vi "Delete row.vi"(10 "tetris block":u8[][](array[numeric])) -> (0 "Rows Deleted":u16, 2 "new tetris block":u8[][](array[numeric]))   [LabVIEW 2018]
panel:
  out "error out":errorcluster
  in  "error in (no error)":errorcluster
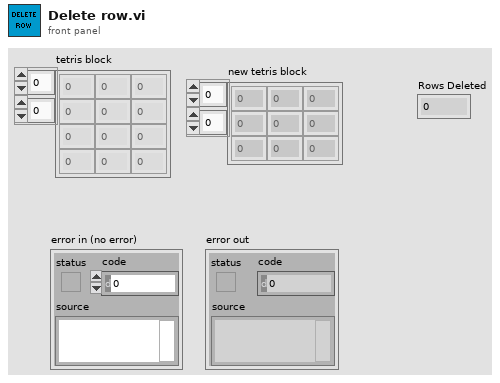
[diagram p1: front panel]
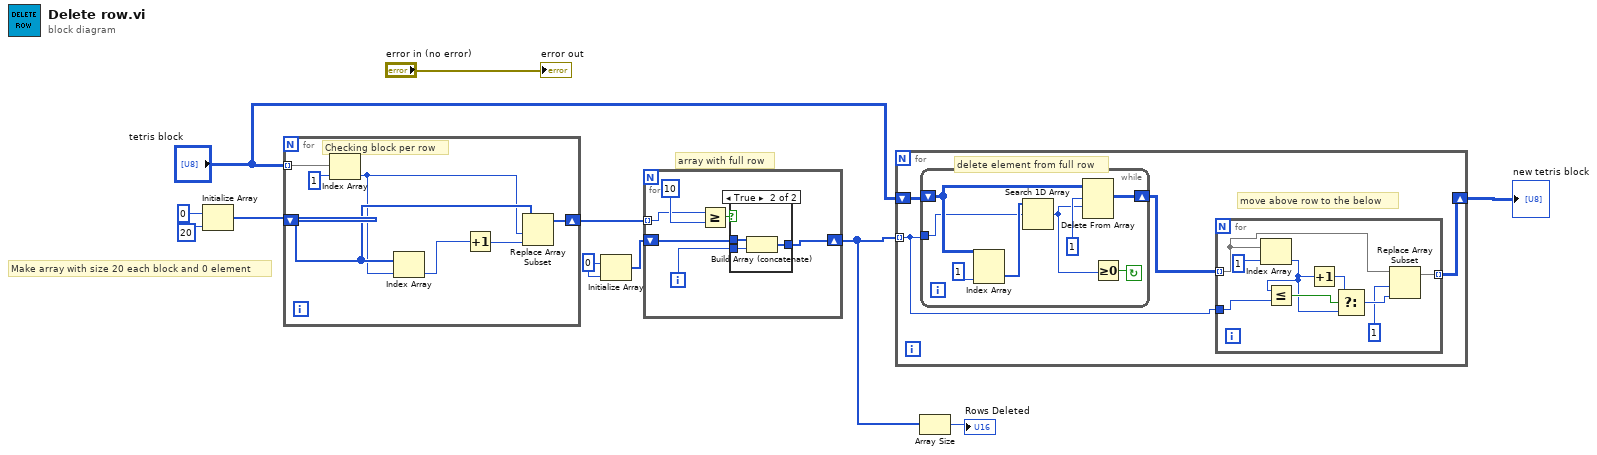
[diagram p0: block diagram]
diagram:
  w5 = 0
  # "array with full row"
  # "Make array with size 20 each block and 0 element"
  n1 = Initialize Array(0, 20) -> (w8:i32[])
  n2 = for {
    tunnel: "tetris block" -> [w14] mode=indexing
    shift-right: [w15] -> w7
    shift-left: w8 -> [w17]
    # "Checking block per row"
    n3 = Index Array(array=w14, index=1) -> (element=w12:u8)
    n4 = Index Array(array=w17, index=w12) -> (element=w18:i32)
    n5 = Increment(x=w18) -> (x+1=w16:i32)
    n6 = Replace Array Subset(array=w17, new element=w16, index=w12) -> (w15:i32[])
  }
  n7 = Initialize Array(w5, w5) -> (w6:i32[])
  n8 = for {
    tunnel: w7 -> [w23] mode=indexing
    shift-right: [w19] -> w1
    shift-left: w6 -> [w21]
    i -> [w20]
    n9 = Greater Or Equal?(x=w23, y=10) -> (x >= y?=w22:bool)
    n10 = case shown="True" w22 {
      tunnel: w21 -> [w25 w28]
      tunnel: w20 -> [_ w27]
      tunnel: [w25 w26] -> w19
      frame False {
      }
      frame True {
        n11 = Build Array (concatenate)(w28, w27) -> (w26:i32[])
      }
    }
  }
  n12 = for {
    shift-right: [w30] -> w3
    shift-left: "tetris block" -> [w32]
    tunnel: w1 -> [w29] mode=indexing
    # "move above row to the below"
    # "delete element from full row"
    n13 = while {
      shift-right: [w44] -> w31
      shift-left: w32 -> [w46]
      tunnel: w29 -> [w42]
      stop <- w47 continue-if-true
      n14 = Index Array(array=w46, index (col)=1) -> (element=w48:u8[])  [unwired: 1 in]
      n15 = Search 1D Array(1D array=w48, element=w42) -> (index of element=w43:i32)  [unwired: 1 in]
      n16 = Delete From Array(array=w46, length=1, index (row)=w43) -> (array with subset deleted=w44:u8[][])  [unwired: 1 in, 1 out]
      n17 = Greater Or Equal To 0?(x=w43) -> (x >= 0?=w47:bool)
    }
    n18 = for {
      tunnel: w31 -> [w34] mode=indexing
      tunnel: w29 -> [w40]
      tunnel: [w33] -> w30 mode=indexing
      n19 = Index Array(array=w34, index=1) -> (element=w37:u8)
      n20 = Less Or Equal?(x=w37, y=w40) -> (x <= y?=w39:bool)
      n21 = Increment(x=w37) -> (x+1=w38:u8)
      n22 = Select(t=w38, s=w39, f=w37) -> (s? t:f=w36:u8)
      n23 = Replace Array Subset(array=w34, new element=w36, index=1) -> (w33:u8[])
    }
  }
  "new tetris block" <- w3
  n24 = Array Size(array=w1) -> (size(s)=→"Rows Deleted":i32)
  "error out" <- "error in (no error)"
